vi "Keithley 6517 Acquire Limit Test.vi"() -> ()   [LabVIEW 2020]
doc: "This example shows how to acquire limit test result of limit 1 or limit2.\n\n<B>Note:</B>\nThis Example is compatible with both model 6517 and 6514."
uses:
  <instrlib>/Keithley 6517/Keithley 6517.lvlib
panel:
  in  "Lower Fail Line 2 (0)":i32
  in  "Upper Fail Line 2 (0)":i32
  in  "Limit Number":i32(ring)=1 items=["Limit1", "Limit2"]
  in  "Upper Limit 2 (1.000000E+0)":dbl=1.0 format="%.6e"
  in  "Lower Limit 2 (-1.000000E+0)":dbl=-1.0 format="%.6e"
  in  "Instrument Model":i32(ring) items=["MODEL 6517B", "MODEL 6517A", "MODEL 6514"]
  in  "Upper Limit 1 (1.000000E+0)":dbl=1.0 format="%.6e"
  in  "Lower Limit 1 (-1.000000E+0)":dbl=-1.0 format="%.6e"
  in  "Lower Fail Line 1 (0)":i32
  in  "Upper Fail Line 1 (0)":i32
  out "Limit2 Test Failed":bool
  out "Limit1 Test Failed":bool
  in  "Limit Number":i32(ring) items=["Limit1", "Limit2"]
  in  "VISA resource name":refnum<visa-resource-name>
  # "(c) 2016-2017 National Instruments.  ALL RIGHTS RESERVED."
  # "Note: This Example is compatible with model 6517 and 6514."
  # "Configure Limit 1"
  # "Configure Limit 2"
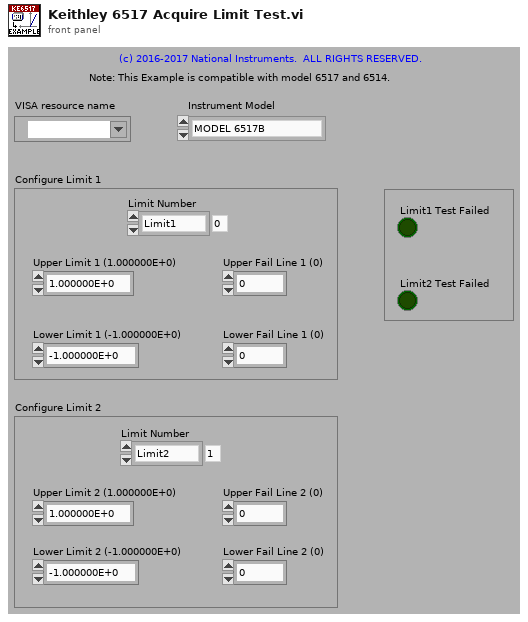
[diagram p1: front panel]
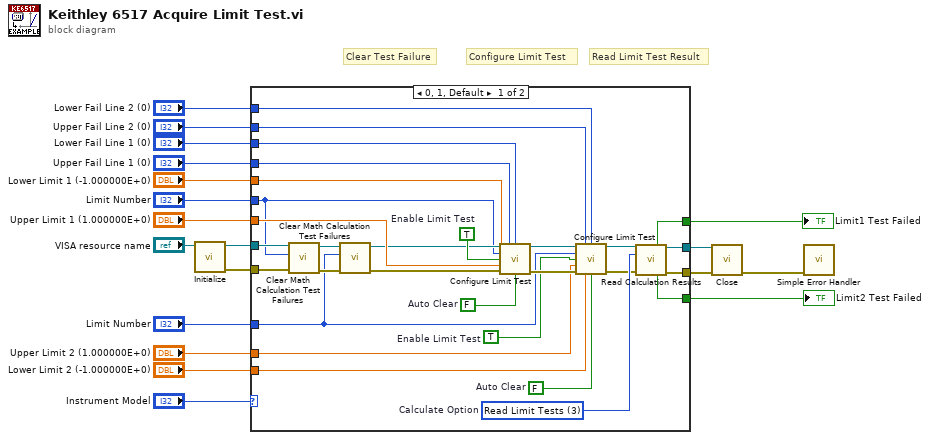
[diagram p0: block diagram]
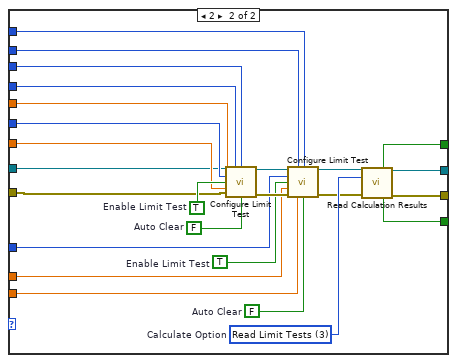
[diagram p2: hidden frame]
diagram:
  # "Read Limit Test Result"
  # "Configure Limit Test"
  # "Clear Test Failure"
  n1 = call <instrlib>:"Initialize.vi"("VISA resource name"="VISA resource name") -> ("error out"=w13:errorcluster, "VISA resource name out"=w14:refnum<visa-resource-name>)  [unwired: 9 in]
  n2 = case shown="0, 1, Default" "Instrument Model" {
    tunnel: [w46 w71] -> w17
    tunnel: "Limit Number" -> [w21 w52]
    tunnel: [w45 w70] -> w15
    tunnel: w14 -> [w26 w49]
    tunnel: w13 -> [w27 w50]
    tunnel: [w44 w69] -> w12
    tunnel: [w43 w68] -> w11
    tunnel: "Upper Fail Line 1 (0)" -> [w42 w67]
    tunnel: "Lower Fail Line 1 (0)" -> [w41 w66]
    tunnel: "Lower Limit 1 (-1.000000E+0)" -> [w40 w65]
    tunnel: "Upper Limit 1 (1.000000E+0)" -> [w39 w64]
    tunnel: "Lower Fail Line 2 (0)" -> [w33 w58]
    tunnel: "Upper Fail Line 2 (0)" -> [w32 w57]
    tunnel: "Lower Limit 2 (-1.000000E+0)" -> [w31 w56]
    tunnel: "Upper Limit 2 (1.000000E+0)" -> [w30 w55]
    tunnel: "Limit Number" -> [w20 w51]
    frame 0, 1, Default {
      w34 = TRUE  # Enable Limit Test
      w35 = FALSE  # Auto Clear
      w38 = 3 items=["Read Math Calculation", "Recalculate Math Calculation", "Read Buffer Data Calculation", "Read Limit Tests"]  # Calculate Option
      w47 = FALSE  # Auto Clear
      w48 = TRUE  # Enable Limit Test
      n3 = call <instrlib>:"Clear Math Calculation Test Failures .vi"("error in (no error)"=w27, "Limit Number (0: Limit1)"=w21, "VISA resource name"=w26) -> ("error out"=w25:errorcluster, "VISA resource name out"=w24:refnum<visa-resource-name>)  [unwired: 7 in]
      n4 = call <instrlib>:"Clear Math Calculation Test Failures .vi"("error in (no error)"=w25, "Limit Number (0: Limit1)"=w20, "VISA resource name"=w24) -> ("error out"=w23:errorcluster, "VISA resource name out"=w22:refnum<visa-resource-name>)  [unwired: 7 in]
      n5 = call <instrlib>:"Configure Limit Test.vi"("VISA resource name"=w22, "Upper Fail Line (0)"=w42, "Lower Fail Line (0)"=w41, "Limit Number (0: Limit1)"=w21, "Enable Limit Test (F: Disable)"=w48, "Upper Limit (1.000000E+0)"=w39, "error in (no error)"=w23, "Lower Limit (-1.000000E+0)"=w40, "Auto Clear (T: Enable)"=w47) -> ("VISA resource name out"=w37:refnum<visa-resource-name>, "error out"=w36:errorcluster)  [unwired: 5 in]
      n6 = call <instrlib>:"Configure Limit Test.vi"("VISA resource name"=w37, "Upper Fail Line (0)"=w32, "Lower Fail Line (0)"=w33, "Limit Number (0: Limit1)"=w20, "Enable Limit Test (F: Disable)"=w34, "Upper Limit (1.000000E+0)"=w30, "error in (no error)"=w36, "Lower Limit (-1.000000E+0)"=w31, "Auto Clear (T: Enable)"=w35) -> ("VISA resource name out"=w28:refnum<visa-resource-name>, "error out"=w29:errorcluster)  [unwired: 5 in]
      n7 = call <instrlib>:"Read Calculation Results.vi"("VISA resource name"=w28, "Calculate Option (0: Read Math Calculation)"=w38, "error in (no error)"=w29) -> ("Limit1 Test Failed"=w46:bool, "VISA resource name out"=w44:refnum<visa-resource-name>, "Limit2 Test Failed"=w45:bool, "error out"=w43:errorcluster)  [unwired: 6 in, 3 out]
    }
    frame 2 {
      w59 = TRUE  # Enable Limit Test
      w60 = FALSE  # Auto Clear
      w63 = 3 items=["Read Math Calculation", "Recalculate Math Calculation", "Read Buffer Data Calculation", "Read Limit Tests"]  # Calculate Option
      w72 = FALSE  # Auto Clear
      w73 = TRUE  # Enable Limit Test
      n8 = call <instrlib>:"Configure Limit Test.vi"("VISA resource name"=w49, "Upper Fail Line (0)"=w67, "Lower Fail Line (0)"=w66, "Limit Number (0: Limit1)"=w52, "Enable Limit Test (F: Disable)"=w73, "Upper Limit (1.000000E+0)"=w64, "error in (no error)"=w50, "Lower Limit (-1.000000E+0)"=w65, "Auto Clear (T: Enable)"=w72) -> ("VISA resource name out"=w62:refnum<visa-resource-name>, "error out"=w61:errorcluster)  [unwired: 5 in]
      n9 = call <instrlib>:"Configure Limit Test.vi"("VISA resource name"=w62, "Upper Fail Line (0)"=w57, "Lower Fail Line (0)"=w58, "Limit Number (0: Limit1)"=w51, "Enable Limit Test (F: Disable)"=w59, "Upper Limit (1.000000E+0)"=w55, "error in (no error)"=w61, "Lower Limit (-1.000000E+0)"=w56, "Auto Clear (T: Enable)"=w60) -> ("VISA resource name out"=w53:refnum<visa-resource-name>, "error out"=w54:errorcluster)  [unwired: 5 in]
      n10 = call <instrlib>:"Read Calculation Results.vi"("VISA resource name"=w53, "Calculate Option (0: Read Math Calculation)"=w63, "error in (no error)"=w54) -> ("Limit1 Test Failed"=w71:bool, "VISA resource name out"=w69:refnum<visa-resource-name>, "Limit2 Test Failed"=w70:bool, "error out"=w68:errorcluster)  [unwired: 6 in, 3 out]
    }
  }
  "Limit1 Test Failed" <- w17
  "Limit2 Test Failed" <- w15
  n11 = call <instrlib>:"Close.vi"("error in (no error)"=w11, "VISA resource name"=w12) -> ("error out"=w18:errorcluster)  [unwired: 9 in]
  n12 = call <vilib>:"Simple Error Handler.vi"("error in (no error)"=w18) -> ()  [unwired: 4 in, 5 out]
